vi "DO Write.vi"(8 "error in (no error)":errorcluster, 10 "Digital Output":bool, 11 "Mech Pump in":refnum<class "Mech Pump.lvclass">) -> (0 "error out":errorcluster)   [LabVIEW 2021, in "Mech Pump.lvlib" / "Mech Pump.lvclass"]
uses:
  Mech Pump.lvclass
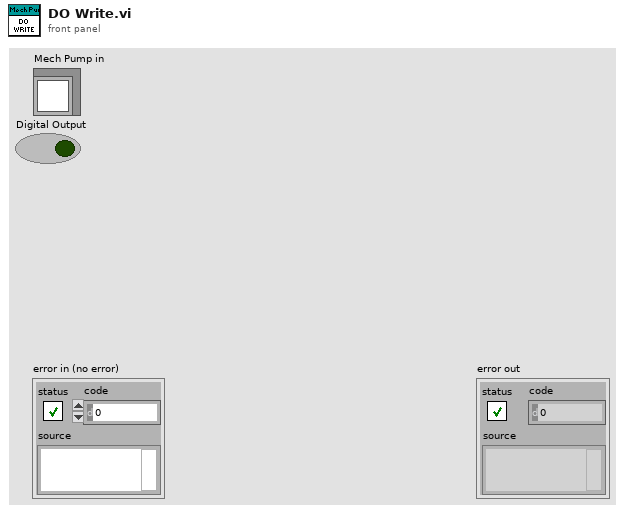
[diagram p1: front panel]
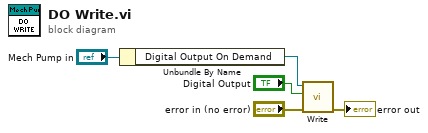
[diagram p0: block diagram]
diagram:
  n1 = Unbundle By Name("Mech Pump in") -> ("Digital Output On Demand"=w4:refnum<class "Digital Output On Demand.lvclass">)
  n2 = call "Write.vi"("error in (no error)"="error in (no error)", "Digital Output"="Digital Output", "Digital Output On Demand in"=w4) -> ("error out"=→"error out":errorcluster)  [unwired: 8 in]
